vi "PAS Server.vi"(11 "PASIn":refnum<class "cPAS.lvclass">) -> ()   [LabVIEW 2015]
uses:
  cPAS.lvclass
  Reusable/Instrument/state.ctl
  Reusable/Instrument/Instrument.lvclass
  Reusable/PAS/Main/PAS.lvclass/PAS.ctl
  Reusable/PAS/Main/Read Freq File.vi
  Reusable/File IO/Class/File Observer.lvclass
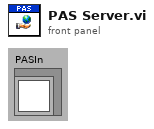
[diagram p1: front panel]
types:
  T1 = typedef "Instrument.lvclass/state.ctl" = enum8{"Configure", "Acquire", "Wait", "Quit", "Handle Error", "NOOP"}
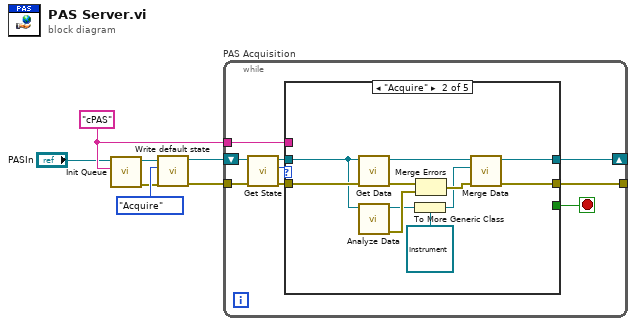
[diagram p0: block diagram]
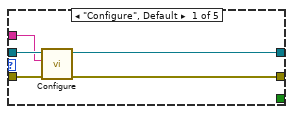
[diagram p2: hidden frame]
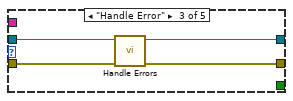
[diagram p3: hidden frame]
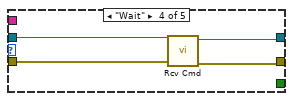
[diagram p4: hidden frame]
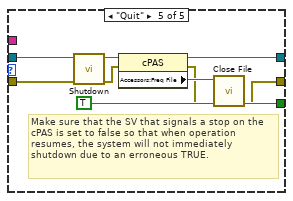
[diagram p5: hidden frame]
diagram:
  w5 = "cPAS" ("queue_name")
  n1 = call "Init Queue.vi"("queue_name"=w5, "Instrument in"="PASIn") -> ("error out"=w2:errorcluster, "Instrument out"=w7:refnum<class "cPAS.lvclass">)  [unwired: 8 in]
  n2 = call "Write default state.vi"("error in (no error)"=w2, "instr state"=state."Acquire", "Instrument in"=w7) -> ("error out"=w1:errorcluster, "Instrument out"=w4:refnum<class "cPAS.lvclass">)  [unwired: 7 in]
  n3 = while "PAS Acquisition" {
    tunnel: w1 -> [w16]
    shift-right: [w10] -> _
    shift-left: w4 -> [w8]
    tunnel: [w14] -> _
    tunnel: w5 -> [w9]
    stop <- w13 stop-if-true
    n4 = call "Get State.vi"("error in"=w16, "Instrument in"=w8) -> ("error out"=w15:errorcluster, "default state"=w12:T1, "Instrument out"=w11:refnum<class "cPAS.lvclass">)  [unwired: 7 in]
    n5 = case shown="\"Acquire\"" w12 {
      tunnel: w11 -> [w21 w31 w36 w40 w48]
      tunnel: w15 -> [w20 w32 w35 w39 w47]
      tunnel: [_ _ _ _ TRUE] -> w13
      tunnel: [w19 w29 w34 w38 w41] -> w10
      tunnel: [w18 w30 w33 w37 w42] -> w14
      tunnel: w9 -> [w17 _ _ _ _]
      frame "Configure", Default {
        n6 = call-dynamic "Configure.vi"("error in"=w20, "name"=w17, "cPAS in"=w21) -> ("error out"=w18:errorcluster, "cPAS out"=w19:refnum<class "cPAS.lvclass">)  [unwired: 7 in]
      }
      frame "Acquire" {
        n7 = call-dynamic "Get Data.vi"("error in"=w32, "cPAS in"=w31) -> ("error out"=w28:errorcluster, "cPAS out"=w26:refnum<class "cPAS.lvclass">)  [unwired: 8 in]
        n8 = call-dynamic "Analyze Data.vi"("cPAS in"=w31) -> ("error out"=w27:errorcluster, "cPAS out"=w22:refnum<class "cPAS.lvclass">)  [unwired: 9 in]
        n9 = To More Generic Class(target class=refnum<class "Instrument.lvclass"> refnum ("Instrument.lvclass"), reference=w22) -> (generic class reference=w23:refnum<class "Instrument.lvclass">)
        n10 = Merge Errors(w28, w27) -> (w25:errorcluster)
        n11 = call-dynamic "Merge Data.vi"("error in"=w25, "Analyzed"=w23, "Acquired"=w26) -> ("error out"=w30:errorcluster, "PAS out"=w29:refnum<class "cPAS.lvclass">)  [unwired: 7 in]
      }
      frame "Handle Error" {
        n12 = call-dynamic "Handle Errors.vi"("error in"=w35, "cPAS in"=w36) -> ("error out"=w33:errorcluster, "cPAS out"=w34:refnum<class "cPAS.lvclass">)  [unwired: 7 in, 1 out]
      }
      frame "Wait" {
        n13 = call-dynamic "Rcv Cmd.vi"("error in"=w39, "cPAS in"=w40) -> ("error out"=w37:errorcluster, "cPAS out"=w38:refnum<class "cPAS.lvclass">)  [unwired: 8 in]
      }
      frame "Quit" {
        # "Make sure that the SV that signals a stop on the cPAS is set to false so that when operation resumes, the system will not immediately shutdown due to an erroneous TRUE."
        n14 = call-dynamic "Shutdown.vi"("error in"=w47, "cPAS in"=w48) -> ("error out"=w45:errorcluster, "cPAS out"=w46:refnum<class "cPAS.lvclass">)  [unwired: 8 in]
        n15 = property class="cPAS"(reference=w46, error in=w45) -> (reference out=w41:refnum<class "cPAS.lvclass">, error out=w43:errorcluster, "Accessors:Freq File"=w44:refnum<class "File Observer.lvclass">)
        n16 = call-dynamic "Close File.vi"("error in"=w43, "File Obs in"=w44) -> ("error out"=w42:errorcluster)  [unwired: 8 in, 1 out]
      }
    }
  }
